vi "PR - Move to relative position.vi"(6 "error in":errorcluster, 7 "Nstep":dbl, 8 "Axis  #":i8=1 min=1 max=6 step=1, 9 "Address / Port":i16=1 min=1 max=31 step=1) -> (0 "error out":errorcluster, 2 "Axis  # dup":i8=1 min=1 max=6 step=1, 3 "Address / Port dup":i16=1 min=1 max=31 step=1)   [LabVIEW 2014]
doc: "Move the motor set on \"Axis#\" of \"Nstep\". The sign of Nstep determines the direction of movement."
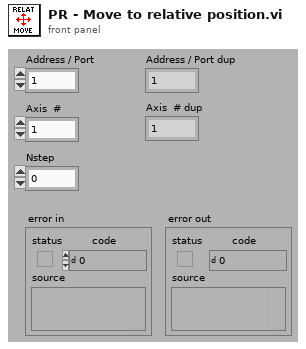
[diagram p1: front panel]
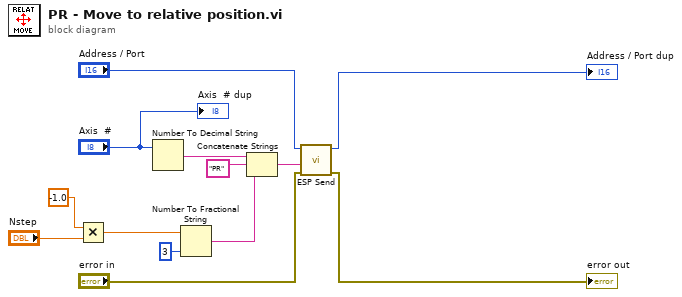
[diagram p0: block diagram]
diagram:
  n1 = Multiply(x=-1.0, y="Nstep") -> (x*y=w2:dbl)
  n2 = Number To Decimal String(number="Axis  #") -> (decimal integer string=w12:string)  [unwired: 1 in]
  n3 = Number To Fractional String(number=w2, precision (6)=i16 3) -> (F-format string=w7:string)  [unwired: 2 in]
  n4 = Concatenate Strings(w12, "PR" ("Substring"), w7) -> (w10:string)
  n5 = call "ESP Send.vi"("error in"="error in", "Command String"=w10, "Address / Port"="Address / Port") -> ("error out"=→"error out":errorcluster, "Address / Port dup"=→"Address / Port dup":i16)  [unwired: 3 in]
  "Axis  # dup" <- "Axis  #"
